vi "party!!!.vi"   [LabVIEW 2012, in "Party_Program.exe.lvrbt"]
uses:
  Party_Program.exe.lvrbt
  <vilib>/NXT/Hardware/Plugins/Tetrix DC Motor/TetrixDCMotorAddress.ctl
  <vilib>/NXT/NXTIO Xnodes/NXTIONodeSubVIs/TETRIX IO Move DC Motors.vi
  <vilib>/NXT/NXTIO Xnodes/NXTIONodeSubVIs/TETRIX IO Stop DC Motors.vi
  <vilib>/NXT/Subs/LVHSConnector.ctl
  <vilib>/NXT/NXTIO Xnodes/AddressXNode/NXTIOAddress.xnode
  <vilib>/NXT/NXTIO Xnodes/NXTIOXNode/NXTIO.xnode
  <vilib>/NXT/LegoClasses/BrickReference/BrickReference.lvclass
types:
  T1 = typedef "TetrixDCMotorAddress.ctl" = i32
  T2 = typedef "LVHSConnector.ctl" = refnum<class "BrickReference.lvclass">
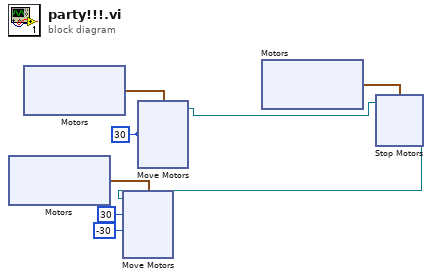
[diagram p0: block diagram]
diagram:
  w5 = i8 30 ("Power/Speed 1")
  n1 = xnode "Motors"() -> ("Motor"=w4:cluster{"TetrixDCMotor":T1, "TetrixDCMotor":T1})
  n2 = xnode "Motors"() -> ("Motor"=w8:cluster{"TetrixDCMotor":T1, "TetrixDCMotor":T1})
  n3 = xnode "Move Motors"("Power/Speed 2"=w5, "Power/Speed 1"=w5, "Motors"=w8) -> ("NXT/EV3"=w6:T2)  [unwired: 1 in]
  n4 = xnode "Motors"() -> ("Motor"=w7:cluster{"TetrixDCMotor":T1, "TetrixDCMotor":T1})
  n5 = xnode "Stop Motors"("Motors"=w7, "NXT/EV3"=w6) -> ("NXT/EV3"=w3:T2)
  n6 = xnode "Move Motors"("Power/Speed 2"=i8 -30, "Power/Speed 1"=i8 30, "Motors"=w4, "NXT/EV3"=w3) -> ()  [unwired: 1 out]
